vi "19.04.2025 class.vi"() -> ()   [LabVIEW 2020]
panel:
  out "deleted portion":dbl[][](array[numeric])
  out "array w/ subset deleted 2":dbl[][](array[numeric])
  out "Array 3":dbl[](array[numeric])
  in  "Array 2":dbl[][](array[numeric])
  out "array w/ subset deleted":dbl[](array[numeric])
  in  "Array":dbl[](array[numeric])
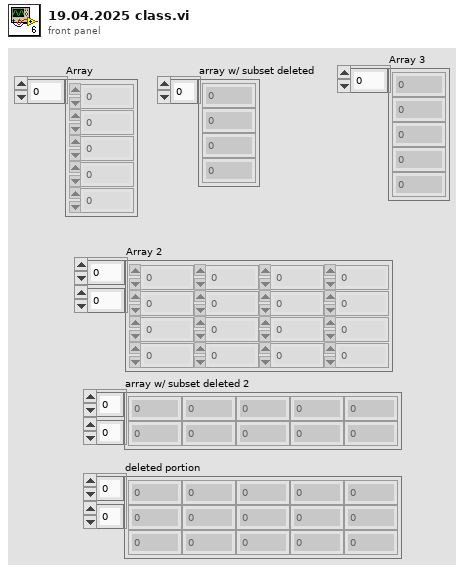
[diagram p1: front panel]
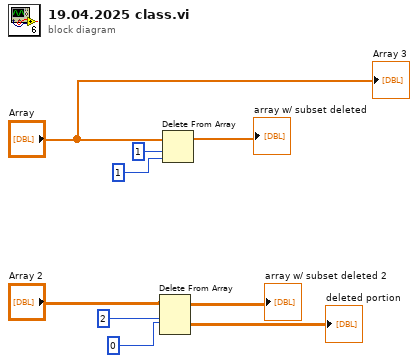
[diagram p0: block diagram]
diagram:
  n1 = Delete From Array "Delete From Array"(array="Array 2", length=2, index (row)=0 ("length")) -> (deleted portion=→"deleted portion":dbl[][], array with subset deleted=→"array w/ subset deleted 2":dbl[][])  [unwired: 1 in]
  n2 = Delete From Array "Delete From Array"(array="Array", length=1, index=1 ("length")) -> (array with subset deleted=→"array w/ subset deleted":dbl[])  [unwired: 1 out]
  "Array 3" <- "Array"
